vi "Create.vi"(8 "error in (no error)":errorcluster, 9 "Outputs":string[](array[string])) -> (0 "error out":errorcluster, 3 "Flip Flop":refnum<class "Flip Flop.lvclass">)   [LabVIEW 2021, in "Flip Flop.lvclass"]
uses:
  Flip Flop.lvclass
  Flip Flop.lvclass/Flip Flop.ctl
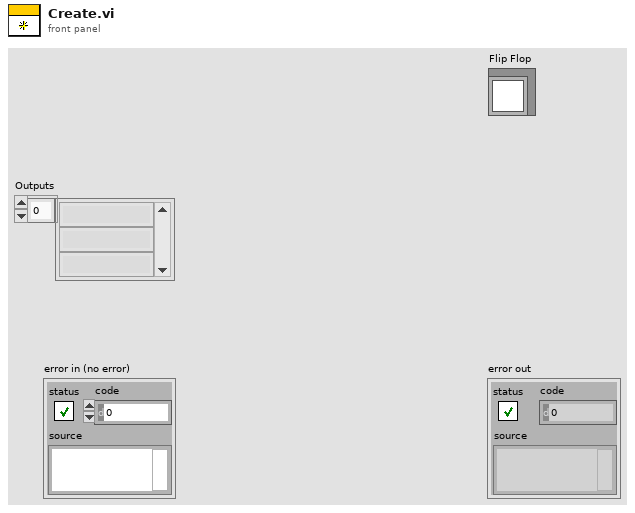
[diagram p1: front panel]
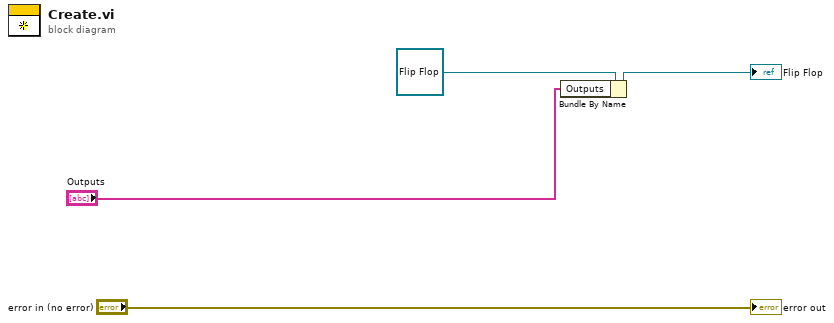
[diagram p0: block diagram]
diagram:
  n1 = Bundle By Name(cluster=refnum<class "Flip Flop.lvclass"> refnum ("Flip Flop"), "Outputs"="Outputs") -> (→"Flip Flop":refnum<class "Flip Flop.lvclass">)
  "error out" <- "error in (no error)"
